vi "Read stop if true.vi"(9 "ForLoop in":refnum<class "ForLoop.lvclass">) -> (3 "ForLoop out":refnum<class "ForLoop.lvclass">, 4 "stop if true":bool)   [LabVIEW 2014, in "Raspberry Pi Compatible Compiler for LabVIEW.lvlib" / "ForLoop.lvclass"]
uses:
  ForLoop.lvclass
  ForLoop.lvclass/ForLoop.ctl
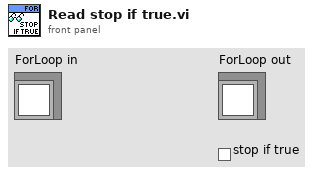
[diagram p1: front panel]
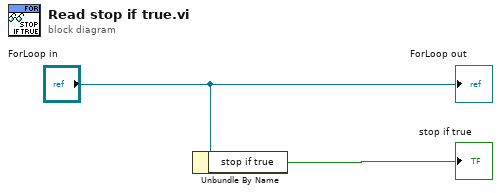
[diagram p0: block diagram]
diagram:
  n1 = Unbundle By Name("ForLoop in") -> ("stop if true"=→"stop if true":bool)
  "ForLoop out" <- "ForLoop in"
